vi "main.vi"() -> ()   [LabVIEW 2013]
uses:
  sub vi/imaging/Image.ctl
  sub vi/gui event/GUI control.ctl
  sub vi/init & communication/Setting-User input.ctl
  <vilib>/Utility/error.llb/DialogType.ctl
  sub vi/imaging/Imaging State.ctl
  sub vi/init & communication/event-package.ctl
  sub vi/init & communication/Event1.ctl
  <vilib>/Analysis/baseanly.llb/Mean (DBL).vi
  <vilib>/Utility/error.llb/Error Cluster From Error Code.vi
  <vilib>/Utility/file.llb/Write To Spreadsheet File (DBL).vi
  <vilib>/ErrorRing/Error Ring.xnode
  <vilib>/Analysis/NI_AALBase.lvlib
panel:
  out "average intensity":dbl(graph)
  out "time per frame (sec)":dbl=0.932688
  out "event loop":i32=10
  out "display loop":i32=341
  in  "Setting User Input":T1={"Image Size\n(pixel * pixel)"=512, "AO Channels"="Dev1/ao0:1", "Y Pos."=0.0, "X Pos."=0.0, "Line surplus\n(pixel)"=150, "Frame surplus\n(us)"=50000, "AI channels"="Dev1/ai0", "Line Number\nper Channel"=32, "Delay Pixel"=10000, "Pixel Dwelling\nTime (us)"=2, "Color Map"=[0, 7171459, 16448250], "head (pixel)"=200, "Zoom (V)"=1.0, "DAQmx Device name"="Dev1", "sample freq (MHz)"=0.5, "angle (deg.)"=0.0} {"Zoom (V)" scale=0.0..1.0; "X Pos." scale=-2.0..2.0; "Y Pos." scale=-2.0..2.0}
  in  "Event Controls":T2={"stop"=FALSE, "save sheet"=FALSE, "Path"=path "D:/Zhiping/ScanImage-LabVIEW/data/20170515_01.tif", "save tiff"=FALSE, "Gain"=1.0, "Offset"=0.0, "save multiple tiffs"=FALSE, "# figs"=10, "saving fig"=path "", "saving"=FALSE} {"Offset" scale=-1.0..1.0; "Gain" scale=1.0..100.0}
  out "Image":T3
  # "选取并移动游标至需要成像的\n中心位置后，会自动设置对应\n的x、y方向中心电压。再次运\n行程序，即可以上次选取的位\n置为中心成像。"
  # "使用步骤：\n1. 设置Setting User Input中的项目。\n2. 运行程序。\n3. 运行时可以调节图像游标、增益、偏置以及\n    文件保存地址，以及使用保存功能。\n（\"ctrl+h\"打开快捷帮助后，鼠标悬停可见各\n    控件的具体帮助）"
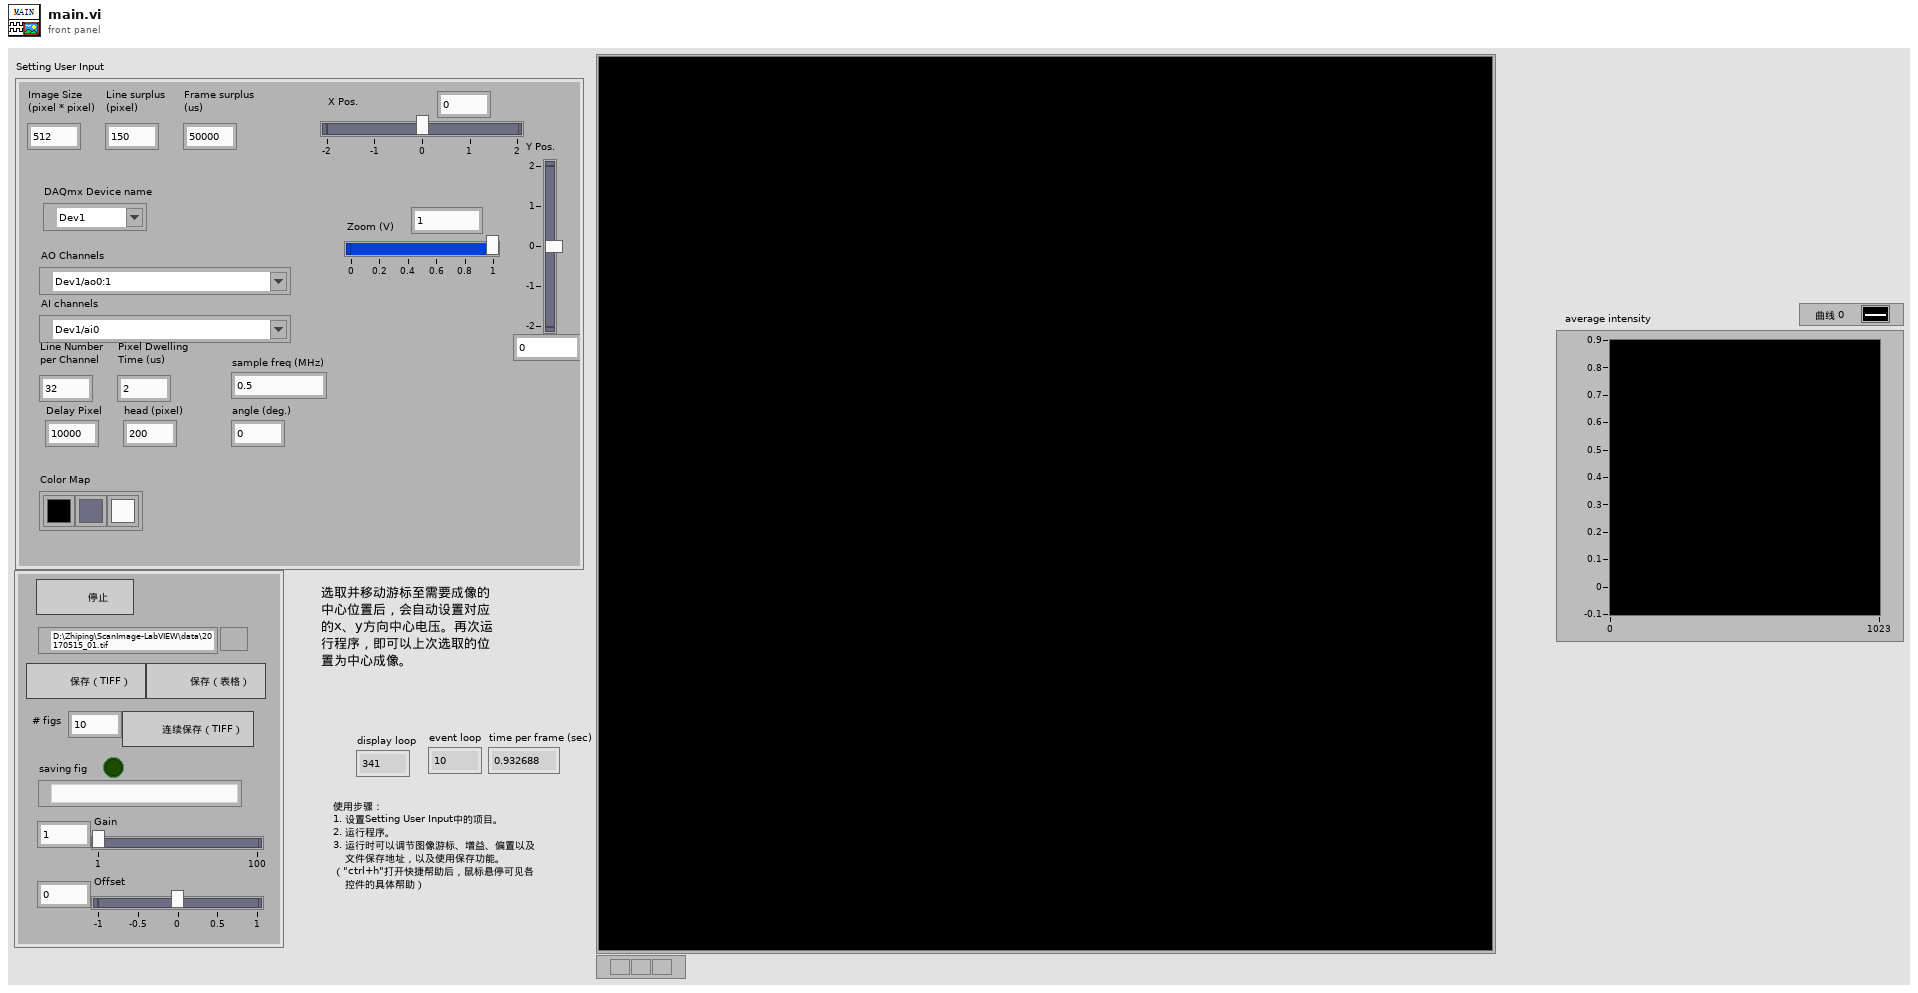
[diagram p1: front panel]
types:
  T1 = typedef "Setting-User input.ctl" = cluster{"Image Size\n(pixel * pixel)":i32, "AO Channels":tag, "Y Pos.":dbl, "X Pos.":dbl, "Line surplus\n(pixel)":i32, "Frame surplus\n(us)":i32, "AI channels":tag, "Line Number\nper Channel":i32, "Delay Pixel":i32, "Pixel Dwelling\nTime (us)":i32, "Color Map":u32[], "head (pixel)":i32, "Zoom (V)":dbl, "DAQmx Device name":tag, "sample freq (MHz)":dbl, "angle (deg.)":dbl}
  T2 = typedef "GUI control.ctl" = cluster{"stop":bool, "save sheet":bool, "Path":path, "save tiff":bool, "Gain":dbl, "Offset":dbl, "save multiple tiffs":bool, "# figs":i32, "saving fig":path, "saving":bool}
  T3 = typedef "Image.ctl" = dbl[][]
  T4 = typedef "Imaging State.ctl" = enum16{"idle", "waiting for saving sheet", "waiting for stopping", "waiting for saving tiff", "init countinuous saving", "continuous saving", ""}
  T5 = typedef "event-package.ctl" = cluster{"Event":T6, "Data":string}
  T6 = typedef "Event1.ctl" = enum16{"null", "stop AI", "stop AO", "stop Imaging", "stop Counter", "save sheet", "restart", "save tiff", "gain/offset changed", "save multiple tiffs"}
  T7 = typedef "DialogType.ctl" = u16
  T8 = typedef "init-status.ctl" = cluster{"Setting":T9, "Event Queue":refnum<queue>, "Data Queue":refnum<queue>, "rendezvous":T10, "CO task out":refnum<k21>, "AO task out":refnum<k21>, "AI task out":refnum<k21>}
  T9 = typedef "Setting.ctl" = cluster{"Image Size\n(pixel * pixel)":i32, "Counter Channel":tag, "Trigger Term":tag, "AO Channels":tag, "Y Pos.":cluster{dbl, dbl}, "X Pos.":cluster{dbl, dbl}, "Line surplus\n(pixel)":i32, "Frame surplus\n(us)":i32, "AI channels":tag, "Line Number\nper Channel":i32, "Delay Pixel":i32, "Pixel Dwelling\nTime (us)":i32, "Color Map":u32[], "head (pixel)":i32, "sample freq (MHz)":dbl, "angle (rad)":dbl}
  T10 = typedef "Rendezvous RefNum" = refnum<k1>
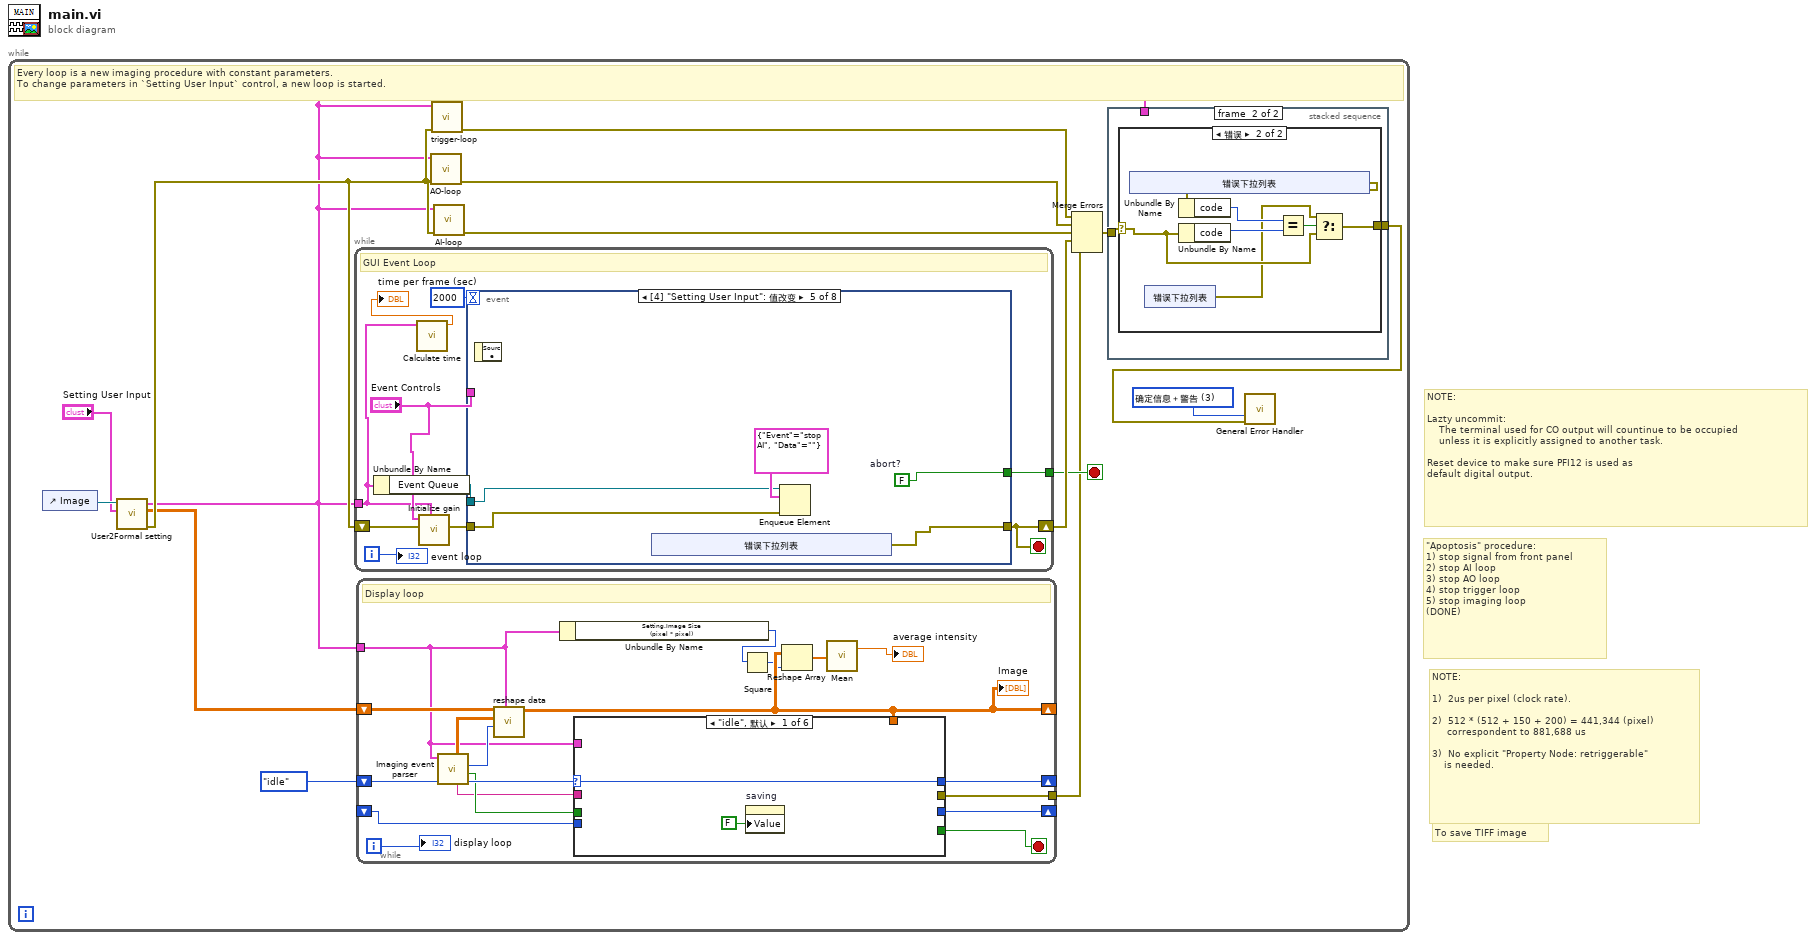
[diagram p0: block diagram]
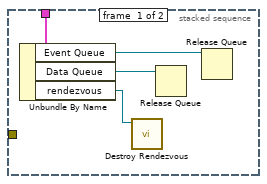
[diagram p2: hidden frame]
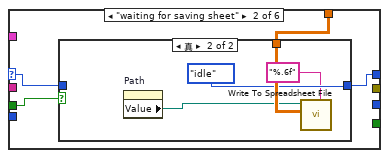
[diagram p4: hidden frame]
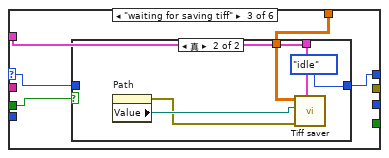
[diagram p6: hidden frame]
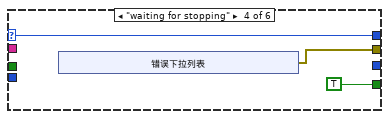
[diagram p8: hidden frame]
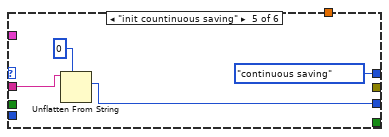
[diagram p9: hidden frame]
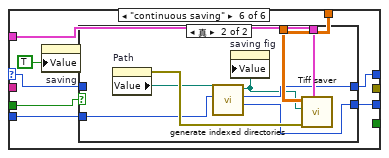
[diagram p10: hidden frame]
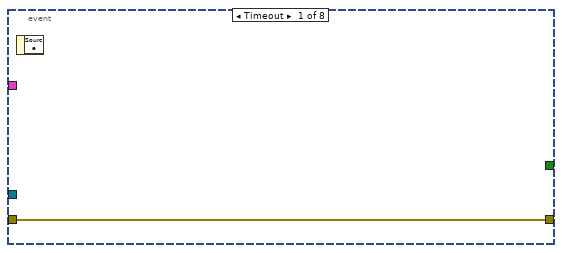
[diagram p12: hidden frame]
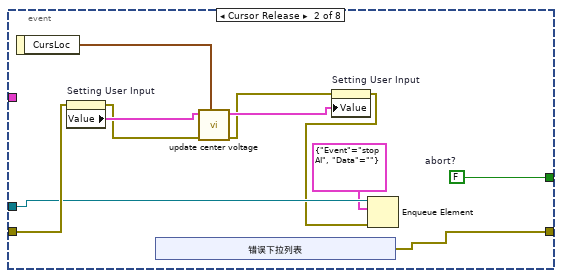
[diagram p13: hidden frame]
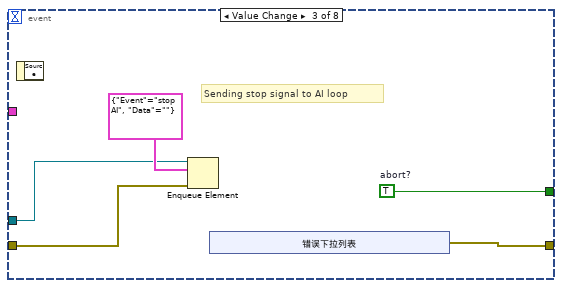
[diagram p14: hidden frame]
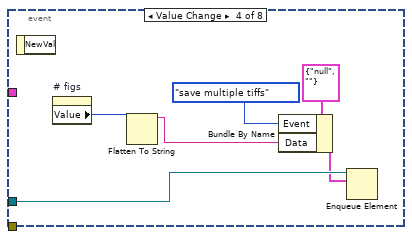
[diagram p15: hidden frame]
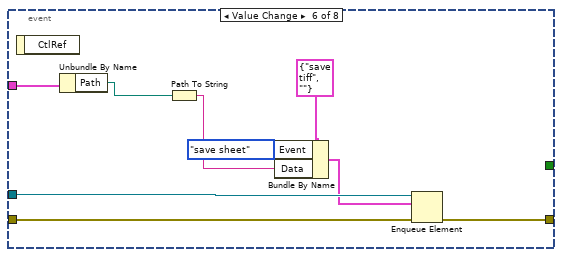
[diagram p16: hidden frame]
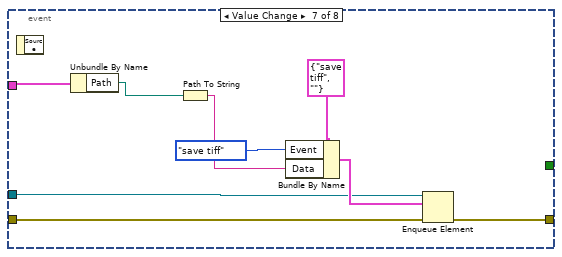
[diagram p17: hidden frame]
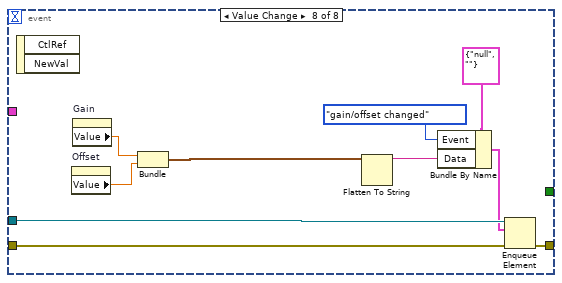
[diagram p18: hidden frame]
diagram:
  # "To save TIFF image"
  # "\"Apoptosis\" procedure:\n1) stop signal from front panel\n2) stop AI loop\n3) stop AO loop\n4) stop trigger loop\n5) stop imaging loop\n(DONE)"
  # "NOTE:\n\nLazty uncommit:\n    The terminal used for CO output will countinue to be occupied\n    unless it is explicitly assigned to another task.\n\nReset device to make sure PFI12 is used as\ndefault digital output."
  # "NOTE:\n\n1)  2us per pixel (clock rate).\n\n2)  512 * (512 + 150 + 200) = 441,344 (pixel)\n     correspondent to 881,688 us\n\n3)  No explicit \"Property Node: retriggerable\"\n    is needed."
  n1 = while {
    stop <- w3 stop-if-true
    w10 = T7 3 items=["无对话框", "确定信息", "继续或停止信息", "确定信息＋警告", "继续/停止+警告"] ("type of dialog (OK msg:1)")
    # "Every loop is a new imaging procedure with constant parameters.\nTo change parameters in `Setting User Input` control, a new loop is started."
    n2 = control-ref of="Image"() -> (w5:refnum<vi>)
    n3 = call "User2Formal setting.vi"("Setting User Input"="Setting User Input", "IntensityGraph输入"=w5) -> ("错误输出"=w15:errorcluster, "Image 2"=w6:T3, "Status"=w1:T8)  [unwired: 7 in]
    n4 = while {
      tunnel: w1 -> [w106]
      shift-right: [w114] -> w14
      shift-left: w15 -> [w111]
      tunnel: [w109] -> w3
      i -> [w108]
      stop <- w114 stop-if-true
      # "GUI Event Loop"
      n5 = Unbundle By Name(w106) -> ("Event Queue"=w112:refnum<queue>)
      n6 = call "Calculate time.vi"("Status"=w106) -> ("数值"=→"time per frame (sec)":dbl)  [unwired: 10 in]
      n7 = call "Initialize gain.vi"("Status"=w106, "错误输入（无错误）"=w111, "Event Controls"="Event Controls") -> ("error out"=w110:errorcluster)  [unwired: 8 in]
      n8 = event shown="[4] \"Setting User Input\": 值改变" {
        selector: _ -> [_ _ _ _ _ _ _ _]
        dyn-events: _ -> [_ _ _ _ _ _ _ _]
        timeout: 2000 -> [_ _ _ _ _ _ _ _]
        tunnel: w110 -> [w115 w121 w132 _ w148 w162 w166 w179]
        tunnel: [w115 w116 w135 _ w146 w161 w165 w178] -> w114
        tunnel: w112 -> [_ w120 w133 w145 w147 w163 w167 w182]
        tunnel: "Event Controls" -> [_ _ _ _ _ w160 w164 _]
        tunnel: [_ w118 w131 _ w150 _ _ _] -> w109
        event Timeout {
          n9 = event-data() -> ()  [unwired: 1 in, 1 out]
        }
        event Cursor Release {
          w118 = FALSE  # abort?
          n10 = event-data() -> ("CursLoc"=w125:cluster{"X":dbl, "Y":dbl})  [unwired: 1 in]
          n11 = property on="Setting User Input" class="Clust (严格)"(error in=w121) -> (error out=w123:errorcluster, "Value"=w124:T1)  [unwired: 1 in, 1 out]
          n12 = xnode "错误下拉列表"() -> ("错误输出"=w116:errorcluster)
          n13 = call "update center voltage.vi"("CursLoc"=w125, "错误输入（无错误）"=w123, "Value in"=w124) -> ("错误输出"=w122:errorcluster, "Value out"=w126:T1)  [unwired: 7 in]
          n14 = property on="Setting User Input" class="Clust (严格)"(error in=w122, "Value"=w126) -> (error out=w117:errorcluster)  [unwired: 1 in, 1 out]
          n15 = Enqueue Element(queue=w120, element=T5 {"Event"=enum."stop AI", "Data"=""} ("元素"), error in (no error)=w117) -> ()  [unwired: 1 in, 3 out]
        }
        event Value Change {
          w131 = TRUE  # abort?
          # "Sending stop signal to AI loop"
          n16 = event-data() -> ()  [unwired: 1 in, 1 out]
          n17 = Enqueue Element(queue=w133, element=T5 {"Event"=enum."stop AI", "Data"=""} ("元素"), error in (no error)=w132) -> ()  [unwired: 1 in, 3 out]
          n18 = xnode "错误下拉列表"() -> ("错误输出"=w135:errorcluster)
        }
        event Value Change {
          n19 = event-data() -> ()  [unwired: 1 in, 1 out]
          n20 = property on="# figs" class="DigNum (严格)"() -> ("Value"=w140:i32)  [unwired: 2 in, 2 out]
          n21 = Flatten To String(anything=w140) -> (data string=w141:string)  [unwired: 3 in, 2 out]
          n22 = Bundle By Name(cluster=T5 {"Event"=enum."null", "Data"=""} ("元素"), "Event"=Event1."save multiple tiffs", "Data"=w141) -> (w143:T5)
          n23 = Enqueue Element(queue=w145, element=w143) -> ()  [unwired: 2 in, 3 out]
        }
        event Value Change {
          w150 = FALSE  # abort?
          n24 = event-data() -> ()  [unwired: 1 in, 1 out]
          n25 = xnode "错误下拉列表"() -> ("错误输出"=w146:errorcluster)
          n26 = Enqueue Element(queue=w147, element=T5 {"Event"=enum."stop AI", "Data"=""} ("元素"), error in (no error)=w148) -> ()  [unwired: 1 in, 3 out]
        }
        event Value Change {
          n27 = event-data() -> ()  [unwired: 1 in, 1 out]
          n28 = Unbundle By Name(w160) -> ("Path"=w158:path)
          n29 = Path To String(path=w158) -> (string=w157:string)
          n30 = Bundle By Name(cluster=T5 {"Event"=enum."save tiff", "Data"=""} ("元素"), "Event"=Event1."save sheet", "Data"=w157) -> (w155:T5)
          n31 = Enqueue Element(queue=w163, element=w155, error in (no error)=w162) -> (error out=w161:errorcluster)  [unwired: 1 in, 2 out]
        }
        event Value Change {
          n32 = event-data() -> ()  [unwired: 1 in, 1 out]
          n33 = Unbundle By Name(w164) -> ("Path"=w171:path)
          n34 = Path To String(path=w171) -> (string=w170:string)
          n35 = Bundle By Name(cluster=T5 {"Event"=enum."save tiff", "Data"=""} ("元素"), "Event"=Event1."save tiff", "Data"=w170) -> (w168:T5)
          n36 = Enqueue Element(queue=w167, element=w168, error in (no error)=w166) -> (error out=w165:errorcluster)  [unwired: 1 in, 2 out]
        }
        event Value Change {
          n37 = event-data() -> ()  [unwired: 1 in, 2 out]
          n38 = property on="Offset" class="Slide (严格)"() -> ("Value"=w173:dbl)  [unwired: 2 in, 2 out]
          n39 = property on="Gain" class="Slide (严格)"() -> ("Value"=w174:dbl)  [unwired: 2 in, 2 out]
          n40 = Bundle("Value"=w174, "Value"=w173) -> (w175:cluster{"Value":dbl, "Value":dbl})  [unwired: 1 in]
          n41 = Flatten To String(anything=w175) -> (data string=w176:string)  [unwired: 3 in, 2 out]
          n42 = Bundle By Name(cluster=T5 {"Event"=enum."null", "Data"=""} ("Event Package"), "Event"=Event1."gain/offset changed", "Data"=w176) -> (w177:T5)
          n43 = Enqueue Element(queue=w182, element=w177, error in (no error)=w179) -> (error out=w178:errorcluster)  [unwired: 1 in, 2 out]
        }
      }
      "event loop" <- w108
    }
    n44 = while {
      tunnel: w1 -> [w38]
      shift-right: [w39] -> _
      shift-left: w6 -> [w48]
      shift-right: [w53] -> _
      shift-left: Imaging_State."idle" -> [w51]
      shift-right: [w43] -> _
      shift-left: _ -> [w42]
      tunnel: [w35] -> w2
      i -> [w45]
      stop <- w52 stop-if-true
      # "Display loop"
      n45 = call "Imaging event parser.vi"("Imaging State in"=w51, "Status"=w38) -> ("Imaging State out"=w50:T4, "last line?"=w49:bool, "line #"=w47:i32, "Data"=w44:string, "Effective lines"=w46:dbl[][])  [unwired: 5 in]
      n46 = call "reshape data.vi"("Status"=w38, "line #"=w47, "Effective lines"=w46, "Image输入"=w48) -> ("Image输出"=w39:T3)  [unwired: 7 in]
      "Image" <- w39
      n47 = Unbundle By Name(w38) -> ("Setting.Image Size\n(pixel * pixel)"=w36:i32)
      n48 = case shown="\"idle\", 默认" w50 {
        selector: w50 -> [w55 w57 w67 w77 _ w92]
        tunnel: w39 -> [_ w59 w69 _ _ w94]
        tunnel: [w55 w56 w66 w77 Imaging_State."continuous saving" ("Imaging State out") w91] -> w53
        tunnel: [_ _ _ TRUE _ _] -> w52
        tunnel: w49 -> [_ w58 w68 _ _ w88]
        tunnel: w38 -> [_ _ w65 _ _ w93]
        tunnel: w44 -> [_ _ _ _ w85 _]
        tunnel: [_ _ _ _ w83 w89] -> w43
        tunnel: w42 -> [_ _ _ _ _ w90]
        tunnel: [_ _ _ w76 _ _] -> w35
        frame "idle", Default {
          n49 = property on="saving" class="Bool (严格)"("Value"=FALSE ("值")) -> ()  [unwired: 2 in, 2 out]
        }
        frame "waiting for saving sheet" {
          n50 = case shown="真" w58 {
            tunnel: w59 -> [_ w64]
            tunnel: w57 -> [w60 _]
            tunnel: [w60 Imaging_State."idle"] -> w56
            frame False {
            }
            frame True {
              n51 = property on="Path" class="Path"() -> ("Value"=w61:path)  [unwired: 2 in, 2 out]
              n52 = call-poly <vilib>:"Write To Spreadsheet File.vi"("format (%.3f)"="%.6f", "2D data"=w64, "file path (dialog if empty)"=w61) -> ()  [unwired: 5 in, 1 out]
            }
          }
        }
        frame "waiting for saving tiff" {
          n53 = case shown="真" w68 {
            tunnel: w69 -> [_ w71]
            tunnel: w67 -> [w70 _]
            tunnel: [w70 Imaging_State."idle"] -> w66
            tunnel: w65 -> [_ w72]
            frame False {
            }
            frame True {
              n54 = property on="Path" class="Path"() -> (error out=w73:errorcluster, "Value"=w74:path)  [unwired: 2 in, 1 out]
              n55 = call "Tiff saver.vi"("Status"=w72, "error in (no error)"=w73, "File Path"=w74, "Image in"=w71) -> ()  [unwired: 7 in, 1 out]
            }
          }
        }
        frame "waiting for stopping" {
          n56 = xnode "错误下拉列表"() -> ("错误输出"=w76:errorcluster)
        }
        frame "init countinuous saving" {
          n57 = Unflatten From String(type=0, binary string=w85) -> (value=w83:i32)  [unwired: 3 in, 2 out]
        }
        frame "continuous saving" {
          n58 = property on="saving" class="Bool (严格)"("Value"=TRUE ("值")) -> ()  [unwired: 2 in, 2 out]
          n59 = case shown="真" w88 {
            tunnel: w94 -> [_ w102]
            tunnel: w92 -> [w96 _]
            tunnel: [w96 w99] -> w91
            tunnel: w93 -> [_ w103]
            tunnel: w90 -> [w95 w100]
            tunnel: [w95 w98] -> w89
            frame False {
            }
            frame True {
              n60 = property on="Path" class="Path"() -> (error out=w104:errorcluster, "Value"=w101:path)  [unwired: 2 in, 1 out]
              n61 = call "generate indexed directories.vi"("image # left in"=w100, "path in"=w101) -> ("image # left out"=w98:i32, "Imaging State out"=w99:T4, "path out"=w97:path)  [unwired: 7 in]
              n62 = property on="saving fig" class="Path"("Value"=w97) -> ()  [unwired: 2 in, 2 out]
              n63 = call "Tiff saver.vi"("Status"=w103, "error in (no error)"=w104, "File Path"=w97, "Image in"=w102) -> ()  [unwired: 7 in, 1 out]
            }
          }
        }
      }
      n64 = Square(x=w36) -> (x^2=w37:i32)
      n65 = Reshape Array(w39, w37) -> (w41:dbl[])
      n66 = call-poly <vilib>:"Mean.vi"("X"=w41) -> ("mean"=→"average intensity":dbl)  [unwired: 1 out]
      "display loop" <- w45
    }
    n67 = call "AO-loop.vi"("错误输入（无错误）"=w15, "Status"=w1) -> ("Error out"=w12:errorcluster)  [unwired: 9 in]
    n68 = call "trigger-loop.vi"("错误输入（无错误）"=w15, "Status"=w1) -> ("error out"=w13:errorcluster)  [unwired: 9 in]
    n69 = call "AI-loop.vi"("错误输入（无错误）"=w15, "Status"=w1) -> ("Error out"=w11:errorcluster)  [unwired: 9 in]
    n70 = Merge Errors(w13, w12, w11, w14, w2) -> (w9:errorcluster)
    n71 = stacked-sequence {
      tunnel: w9 -> [_ w21]
      tunnel: [_ w20] -> w8
      tunnel: w1 -> [w19 _]
      frame #0 {
        n72 = Unbundle By Name(w19) -> ("Event Queue"=w18:refnum<queue>, "Data Queue"=w17:refnum<queue>, "rendezvous"=w16:T10)
        n73 = call <vilib>:"Destroy Rendezvous.vi"("rendezvous"=w16) -> ()  [unwired: 5 in, 2 out]
        n74 = Release Queue(queue=w17) -> ()  [unwired: 2 in, 3 out]
        n75 = Release Queue(queue=w18) -> ()  [unwired: 2 in, 3 out]
      }
      frame #1 {
        n76 = case shown="错误" w21 {
          selector: w21 -> [w22 w25]
          tunnel: [w22 w23] -> w20
          frame No Error {
          }
          frame Error {
            n77 = xnode "错误下拉列表"() -> ("错误输出"=w28:errorcluster)
            n78 = xnode "错误下拉列表"() -> ("错误输出"=w24:errorcluster)
            n79 = Unbundle By Name(w28) -> ("code"=w27:i32)
            n80 = Unbundle By Name(w25) -> ("code"=w26:i32)
            n81 = Equal?(x=w27, y=w26) -> (x = y?=w29:bool)
            n82 = Select(t=w24, s=w29, f=w25) -> (s? t:f=w23:errorcluster)
          }
        }
      }
    }
    n83 = call <vilib>:"General Error Handler.vi"("type of dialog (OK msg:1)"=w10, "error in (no error)"=w8) -> ()  [unwired: 9 in, 5 out]
  }
